vi "Averaged DC-RMS for N Chan.vi"(6 "averaging control":T2={"window for DC"=enum."Rectangular (none)", "output function"=enum."DC and RMS", "window for RMS"=enum."Rectangular (none)", "exp. time constant"=-1.0, "Ignore input start time"=FALSE} {"exp. time constant" format="%0.2p"}, 7 "reset":bool, 8 "error in (no error)":errorcluster, 9 "averaging time":dbl=-1.0 format="%0.2p", 10 "averaging type":enum16{"Linear", "Exponential"}(ring), 11 "signals in":waveform(dbl)[](array[waveform])) -> (0 "error out":errorcluster, 2 "RMS value waveforms":waveform(dbl)[](array[waveform]), 3 "DC value waveforms":waveform(dbl)[](array[waveform]), 4 "measurements info":T1(array[cluster]) {"uncertainty" format="%0.2p"}, 5 "data ready":bool)   [LabVIEW 2020, in "NI_MAPro.lvlib"]
doc: "Calculates the DC and RMS values of an input waveform or array of waveforms. This VI is similar to the Basic Averaged DC-RMS VI, but this VI gives more precise control over the individual DC and RMS calculations."
uses:
  NI_MAPro.lvlib
  NI_MABase.lvlib
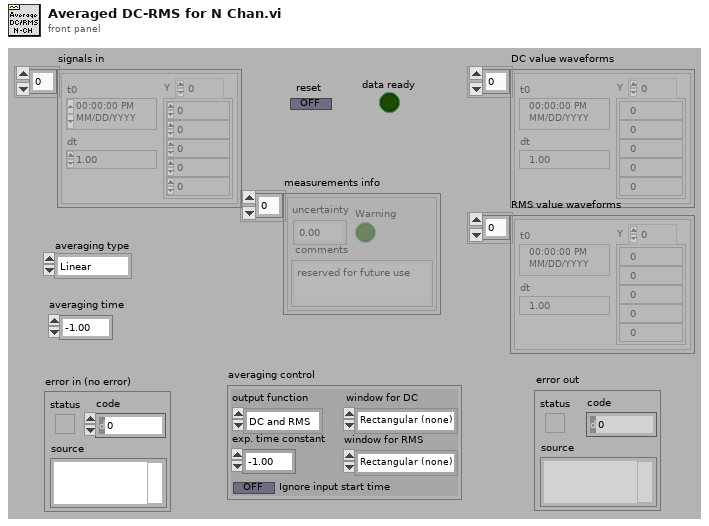
[diagram p1: front panel]
types:
  T1 = cluster{"uncertainty":dbl, "Warning":bool, "comments":string}[]
  T2 = cluster{"window for DC":enum16{"Rectangular (none)", "Hanning", "Low side lobe"}, "output function":enum16{"DC only", "RMS only", "DC and RMS"}, "window for RMS":enum16{"Rectangular (none)", "Hanning", "Low side lobe"}, "exp. time constant":dbl, "Ignore input start time":bool}
  T3 = cluster{"DC history":dbl, "RMS history":dbl, "exp TC (samples)":dbl, "buffer size":i32, "t0 history":timestamp, "dt history":dbl, "timestamp":timestamp, "buffer":dbl[]}
  T4 = cluster{"uncertainty":dbl, "Warning":bool, "comments":string}
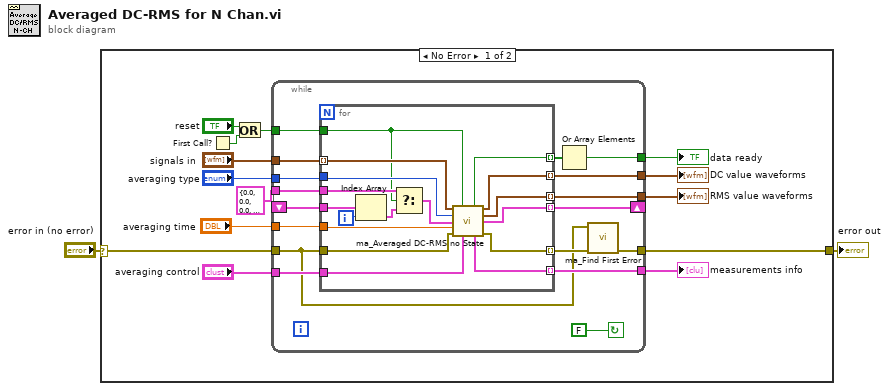
[diagram p0: block diagram]
diagram:
  n1 = case shown="No Error" "error in (no error)" {
    selector: "error in (no error)" -> [w4 w51]
    tunnel: [w5 w51] -> w2
    frame No Error {
      n2 = First Call?() -> (First Call?: T/F=w13:bool)
      n3 = Or(x="reset", y=w13) -> (x .or. y?=w12:bool)
      n4 = while {
        tunnel: [w20] -> w6
        tunnel: "averaging control" -> [w25]
        tunnel: T3 {"DC history"=0.0, "RMS history"=0.0, "exp TC (samples)"=0.0, "buffer size"=0, "t0 history"=timestamp(0 s since 1904-01-01), "dt history"=0.0, "timestamp"=timestamp(0 s since 1904-01-01), "buffer"=[]} ("state info") -> [w21]
        shift-left: _ -> [w22]
        shift-right: [w28] -> _
        tunnel: w4 -> [w17]
        tunnel: "averaging type" -> [w33]
        tunnel: [w26] -> w8
        tunnel: "signals in" -> [w24]
        tunnel: "averaging time" -> [w30]
        tunnel: [w31] -> w16
        tunnel: [w32] -> w15
        tunnel: w12 -> [w23]
        tunnel: [w18] -> w5
        stop <- FALSE continue-if-true
        n5 = for {
          tunnel: w33 -> [w49]
          tunnel: [w42] -> w32 mode=indexing
          tunnel: [w43] -> w31 mode=indexing
          tunnel: w30 -> [w47]
          tunnel: w24 -> [w48] mode=indexing
          tunnel: [w44] -> w29 mode=indexing
          tunnel: w22 -> [w37]
          tunnel: [w50] -> w28 mode=indexing
          tunnel: w23 -> [w35]
          tunnel: w25 -> [w41]
          tunnel: w21 -> [w36]
          tunnel: [w34] -> w20 mode=indexing
          tunnel: w17 -> [w46]
          tunnel: [w45] -> w19 mode=indexing
          i -> [w39]
          n6 = Index Array(array=w37, index=w39) -> (element=w40:T3)
          n7 = Select(t=w36, s=w35, f=w40) -> (s? t:f=w38:T3)
          n8 = call "ma_Averaged DC-RMS no State.vi"("signal in"=w48, "reset"=w35, "averaging type"=w49, "state info"=w38, "averaging time"=w47, "error in"=w46, "averaging control"=w41) -> ("data ready"=w44:bool, "DC value waveform"=w43:waveform(dbl), "RMS value waveform"=w42:waveform(dbl), "state info"=w50:T3, "measurement info cluster"=w34:T4, "error out"=w45:errorcluster)  [unwired: 3 in]
        }
        n9 = Or Array Elements(Boolean array=w29) -> (logical OR=w26:bool)
        n10 = call "ma_Find First Error.vi"("error array in"=w19, "error in 1 (no error)"=w17) -> ("error out"=w18:errorcluster)  [unwired: 5 in]
      }
      "data ready" <- w8
      "DC value waveforms" <- w16
      "RMS value waveforms" <- w15
      "measurements info" <- w6
    }
    frame Error {
    }
  }
  "error out" <- w2
